vi "Server_min.vi"   [LabVIEW 2014]
uses:
  CRD/nCRD.lvclass
  Reusable/Instrument/state.ctl
  Devices/Alicat/Session Based/Alicat Device.lvclass
  Reusable/Instrument/Instrument.lvclass
types:
  T1 = typedef "Instrument.lvclass/state.ctl" = enum8{"Configure", "Acquire", "Wait", "Quit", "Handle Error", "NOOP"}
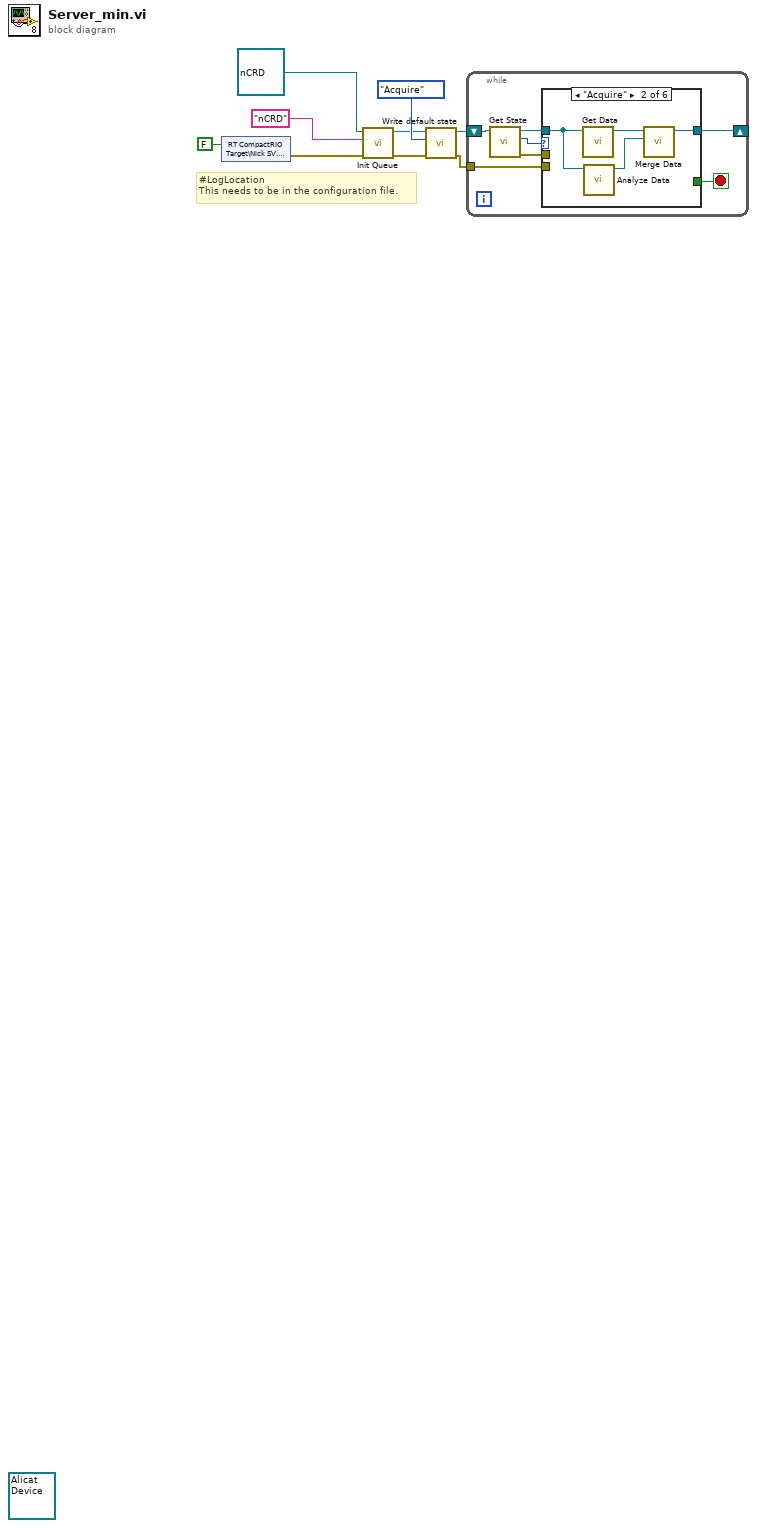
[diagram p0: block diagram]
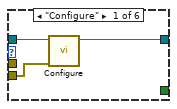
[diagram p2: hidden frame]
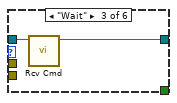
[diagram p3: hidden frame]
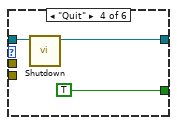
[diagram p4: hidden frame]
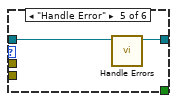
[diagram p5: hidden frame]
diagram:
  (unwired) refnum<class "Alicat Device.lvclass"> refnum ("Alicat Device")
  # "#LogLocation\nThis needs to be in the configuration file."
  n1 = shared-variable "RT CompactRIO Target\\Nick SV.lvlib\\Stop"(FALSE ("Stop")) -> (error out=w8:errorcluster)  [unwired: 1 in]
  n2 = call "Init Queue.vi"("error in"=w8, "queue_name"="nCRD", "Instrument in"=refnum<class "nCRD.lvclass"> refnum ("nCRD")) -> ("error out"=w3:errorcluster, "Instrument out"=w4:refnum<class "nCRD.lvclass">)  [unwired: 7 in]
  n3 = call "Write default state.vi"("error in (no error)"=w3, "instr state"=state."Acquire", "Instrument in"=w4) -> ("error out"=w5:errorcluster, "Instrument out"=w6:refnum<class "nCRD.lvclass">)  [unwired: 7 in]
  n4 = while {
    shift-right: [w12] -> _
    shift-left: w6 -> [w13]
    tunnel: w5 -> [w11]
    stop <- w15 stop-if-true
    n5 = call "Get State.vi"("Instrument in"=w13) -> ("error out"=w10:errorcluster, "default state"=w16:T1, "Instrument out"=w14:refnum<class "nCRD.lvclass">)  [unwired: 8 in]
    n6 = case shown="\"Acquire\"" w16 {
      tunnel: [_ _ _ TRUE _ _] -> w15
      tunnel: w14 -> [w19 w23 w25 w27 w30 w31]
      tunnel: [w18 w22 w24 w26 w29 w31] -> w12
      tunnel: w11 -> [w17 _ _ _ _ _]
      tunnel: w10 -> [_ _ _ _ _ _]
      frame "Configure" {
        n7 = call-dynamic "Configure.vi"("error in"=w17, "nCRD in"=w19) -> ("nCRD out"=w18:refnum<class "nCRD.lvclass">)  [unwired: 8 in, 1 out]
      }
      frame "Acquire" {
        n8 = call-dynamic "Get Data.vi"("nCRD in"=w23) -> ("nCRD out"=w21:refnum<class "nCRD.lvclass">)  [unwired: 9 in, 1 out]
        n9 = call-dynamic "Analyze Data.vi"("nCRD in"=w23) -> ("nCRD out"=w20:refnum<class "nCRD.lvclass">)  [unwired: 9 in, 1 out]
        n10 = call-dynamic "Merge Data.vi"("Analyzed"=w20, "Acquired"=w21) -> ("CRDS out"=w22:refnum<class "nCRD.lvclass">)  [unwired: 8 in, 1 out]
      }
      frame "Wait" {
        n11 = call-dynamic "Rcv Cmd.vi"("nCRD in"=w25) -> ("nCRD out"=w24:refnum<class "nCRD.lvclass">)  [unwired: 9 in, 1 out]
      }
      frame "Quit" {
        n12 = call-dynamic "Shutdown.vi"("nCRD in"=w27) -> ("nCRD out"=w26:refnum<class "nCRD.lvclass">)  [unwired: 9 in, 1 out]
      }
      frame "Handle Error" {
        n13 = call-dynamic "Handle Errors.vi"("nCRD in"=w30) -> ("nCRD out"=w29:refnum<class "nCRD.lvclass">)  [unwired: 8 in, 2 out]
      }
      frame "NOOP", Default {
      }
    }
  }
